vi "Vision Processing.vi"(4 "error in (no error)":errorcluster) -> ()   [LabVIEW 2015]
uses:
  Vision Support Code/Camera Types.ctl
  <vilib>/Rock Robotics/WPI/Camera/WPI_CameraImageSize.ctl
  <vilib>/Rock Robotics/WPI/Camera/WPI_CameraWhite Balance Values.ctl
  <vilib>/Rock Robotics/WPI/Camera/WPI_CameraExposure Values.ctl
  <vilib>/Rock Robotics/WPI/Camera/WPI_CameraFrameRate.ctl
  Robot Global Data.vi
  <vilib>/vision/NI_Vision_Development_Module.lvlib
panel:
  in  "Image Size":T1=enum."320x240"
  in  "Image Size 2":T1=enum."320x240"
  out "Highest Aspect":dbl=-1.0
  out "Target 2":bool
  out "Target 1":bool
  in  "Center Threshold":dbl=0.1
  out "Target 0":bool
  out "Highest Avg Score":dbl
  in  "Min Score Threshold":i32=75
  out "Detected Targets":T2(array[cluster]) {"Normalized Rect"."Numeric 5" format="%#_2g"; "Normalized Rect"."Numeric 3" format="%#_2g"; "Normalized Rect"."Numeric 2" format="%#_2g"; "Normalized Rect"."Numeric" format="%#_2g"}
  out "Sorted Particle Scores":T3(array[cluster]) {"Moment Factor" format="%#_3g"; "Aspect Ratio" format="%#_3g"; "Area to CH" format="%#_3g"; "X" format="%#_3g"; "Y" format="%#_3g"}
  in  "Display Original":bool
  in  "Display Mask":bool
  out "fps":dbl
  in  "Emphasize Limit Tests":bool
  in  "Camera Type":T4=enum."MS HD3000 square"
  in  "Aspect Fudge Factor":dbl=1.0
  in  "Score Threshold":dbl=75.0
  out "ms to process":u32
  out "Qualified Particles":i32
  in  "LED Color":T5={"Hue"={17.898766599709568, 122.67388403082947}, "Sat"={24.285714285714295, 255.0}, "Val"={145.71428571428572, 255.0}} {"Hue" scale=0.0..255.0 scale format="%#_3g"}
  out "Masked":T6(plugin-control)
  out "Original Image":T6(plugin-control)
  # "This is only the initial camera size.\nOther camera setup is done\non the diagram. Notice it is set\nonce before the loop but can be\nupdated within the loop if needed."
  # "Instructions:\nUse LED Color to threshold and build particles. Adjust calibration if needed.\nDisplays are very useful for debugging, but will slow down execution, so you\nmay want to disable once working.\nAnnotations show the rectangle and the scores from top to bottom.\nChange camera setting on diagram."
  # "Density Profile"
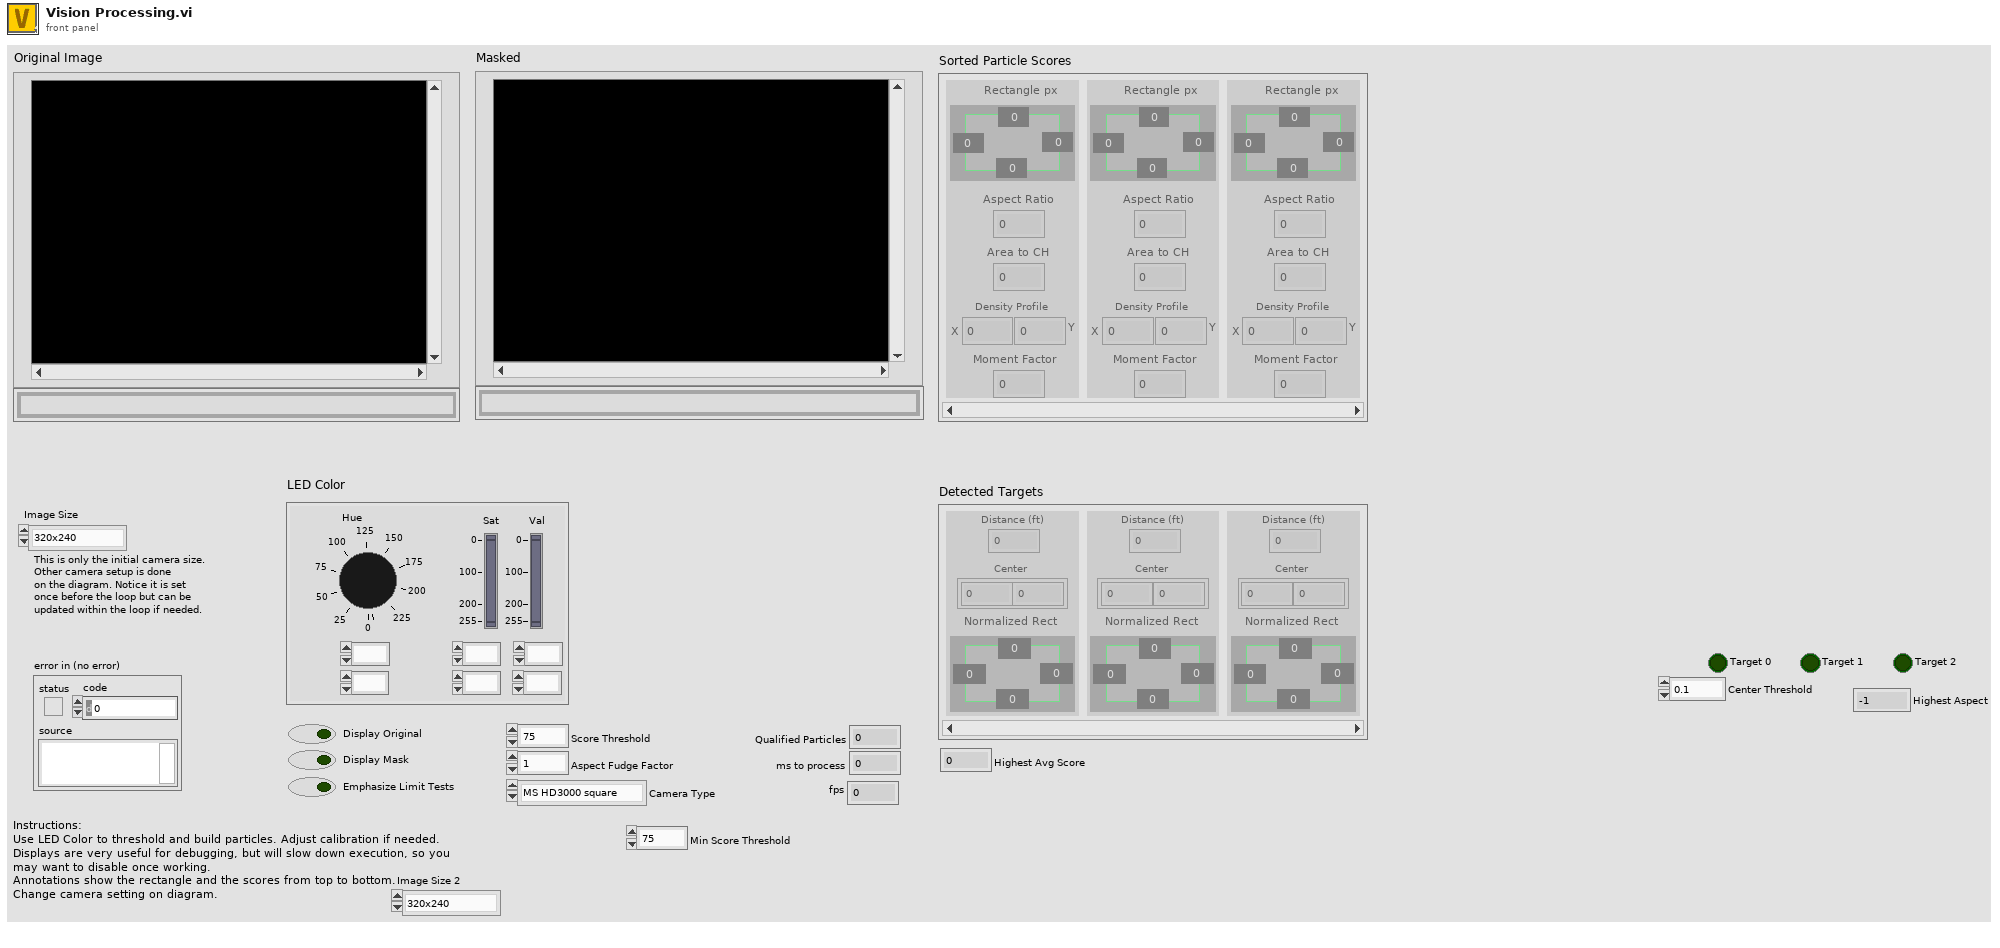
[diagram p1: front panel]
types:
  T1 = typedef "WPI_CameraImageSize.ctl" = enum16{"640x480", "320x240", "160x120", "Custom"}
  T2 = cluster{"Distance (ft)":dbl, "Center":cluster{dbl, dbl}, "Normalized Rect":cluster{"Numeric":dbl, "Numeric 2":dbl, "Numeric 3":dbl, "Numeric 5":dbl}}[]
  T3 = cluster{"Rectangle px":cluster{"Numeric":dbl, "Numeric 2":dbl, "Numeric 3":dbl, "Numeric 5":dbl}, "Aspect Ratio":dbl, "Area to CH":dbl, "X":dbl, "Y":dbl, "Moment Factor":dbl}[]
  T4 = typedef "Camera Types.ctl" = enum16{"206", "1011", "1013", "MS HD3000 square", "MS HD3000 640x480"}
  T5 = cluster{"Hue":cluster{dbl, dbl}, "Sat":cluster{dbl, dbl}, "Val":cluster{dbl, dbl}}
  T6 = typedef "IMAQ Image.ctl" = refnum<image>
  T7 = typedef "WPI_CameraFrameRate.ctl" = u32
  T8 = typedef "WPI_CameraWhite Balance Values.ctl" = enum16{"Auto", "Fixed indoor", "Fixed outdoor 1", "Fixed outdoor 2", "Fixed fluorescent 1", "Fixed fluorescent 2", "Hold current", "Custom"}
  T9 = typedef "WPI_CameraExposure Values.ctl" = enum16{"Auto", "Flicker-free 50 Hz", "Flicker-free 60 Hz", "Hold current", "Custom"}
  T10 = typedef "Particle Parameters" = i32
  T11 = typedef "Image Type" = u32
  T12 = typedef "WPI_CameraDevRef.ctl" = cluster{"Camera Address":string, "CameraStatus":errorcluster}
  T13 = cluster{"Bounding box":cluster{"left":dbl, "top":dbl, "right":dbl, "bottom":dbl}, "Aspect Ratio":dbl, "Area to CH":dbl, "X Mask":dbl, "Y Mask":dbl, "Moment":dbl}[]
  T14 = cluster{"Rectangle":cluster{"Numeric":dbl, "Numeric 2":dbl, "Numeric 3":dbl, "Numeric 5":dbl}, "L":dbl, "Area to CH":dbl, "X":dbl, "Y":dbl, "Moment Factor":dbl}[]
  T15 = cluster{"Sorted Scores[0]":cluster{"Rectangle":cluster{"Numeric":dbl, "Numeric 2":dbl, "Numeric 3":dbl, "Numeric 5":dbl}, "L":dbl, "Area to CH":dbl, "X":dbl, "Y":dbl, "Moment Factor":dbl}, "Sorted Scores[1]":cluster{"Rectangle":cluster{"Numeric":dbl, "Numeric 2":dbl, "Numeric 3":dbl, "Numeric 5":dbl}, "L":dbl, "Area to CH":dbl, "X":dbl, "Y":dbl, "Moment Factor":dbl}, "Sorted Scores[2]":cluster{"Rectangle":cluster{"Numeric":dbl, "Numeric 2":dbl, "Numeric 3":dbl, "Numeric 5":dbl}, "L":dbl, "Area to CH":dbl, "X":dbl, "Y":dbl, "Moment Factor":dbl}, "Sorted Scores[3]":cluster{"Rectangle":cluster{"Numeric":dbl, "Numeric 2":dbl, "Numeric 3":dbl, "Numeric 5":dbl}, "L":dbl, "Area to CH":dbl, "X":dbl, "Y":dbl, "Moment Factor":dbl}, "Sorted Scores[4]":cluster{"Rectangle":cluster{"Numeric":dbl, "Numeric 2":dbl, "Numeric 3":dbl, "Numeric 5":dbl}, "L":dbl, "Area to CH":dbl, "X":dbl, "Y":dbl, "Moment Factor":dbl}, "Sorted Scores[5]":cluster{"Rectangle":cluster{"Numeric":dbl, "Numeric 2":dbl, "Numeric 3":dbl, "Numeric 5":dbl}, "L":dbl, "Area to CH":dbl, "X":dbl, "Y":dbl, "Moment Factor":dbl}, "Sorted Scores[6]":cluster{"Rectangle":cluster{"Numeric":dbl, "Numeric 2":dbl, "Numeric 3":dbl, "Numeric 5":dbl}, "L":dbl, "Area to CH":dbl, "X":dbl, "Y":dbl, "Moment Factor":dbl}, "Sorted Scores[7]":cluster{"Rectangle":cluster{"Numeric":dbl, "Numeric 2":dbl, "Numeric 3":dbl, "Numeric 5":dbl}, "L":dbl, "Area to CH":dbl, "X":dbl, "Y":dbl, "Moment Factor":dbl}, "Sorted Scores[8]":cluster{"Rectangle":cluster{"Numeric":dbl, "Numeric 2":dbl, "Numeric 3":dbl, "Numeric 5":dbl}, "L":dbl, "Area to CH":dbl, "X":dbl, "Y":dbl, "Moment Factor":dbl}}
  T16 = cluster{"Found Targets[0]":cluster{"Distance (ft)":dbl, "Center":cluster{dbl, dbl}, "Normalized Rect":cluster{"Numeric":dbl, "Numeric 2":dbl, "Numeric 3":dbl, "Numeric 5":dbl}}, "Found Targets[1]":cluster{"Distance (ft)":dbl, "Center":cluster{dbl, dbl}, "Normalized Rect":cluster{"Numeric":dbl, "Numeric 2":dbl, "Numeric 3":dbl, "Numeric 5":dbl}}, "Found Targets[2]":cluster{"Distance (ft)":dbl, "Center":cluster{dbl, dbl}, "Normalized Rect":cluster{"Numeric":dbl, "Numeric 2":dbl, "Numeric 3":dbl, "Numeric 5":dbl}}, "Found Targets[3]":cluster{"Distance (ft)":dbl, "Center":cluster{dbl, dbl}, "Normalized Rect":cluster{"Numeric":dbl, "Numeric 2":dbl, "Numeric 3":dbl, "Numeric 5":dbl}}, "Found Targets[4]":cluster{"Distance (ft)":dbl, "Center":cluster{dbl, dbl}, "Normalized Rect":cluster{"Numeric":dbl, "Numeric 2":dbl, "Numeric 3":dbl, "Numeric 5":dbl}}, "Found Targets[5]":cluster{"Distance (ft)":dbl, "Center":cluster{dbl, dbl}, "Normalized Rect":cluster{"Numeric":dbl, "Numeric 2":dbl, "Numeric 3":dbl, "Numeric 5":dbl}}, "Found Targets[6]":cluster{"Distance (ft)":dbl, "Center":cluster{dbl, dbl}, "Normalized Rect":cluster{"Numeric":dbl, "Numeric 2":dbl, "Numeric 3":dbl, "Numeric 5":dbl}}, "Found Targets[7]":cluster{"Distance (ft)":dbl, "Center":cluster{dbl, dbl}, "Normalized Rect":cluster{"Numeric":dbl, "Numeric 2":dbl, "Numeric 3":dbl, "Numeric 5":dbl}}, "Found Targets[8]":cluster{"Distance (ft)":dbl, "Center":cluster{dbl, dbl}, "Normalized Rect":cluster{"Numeric":dbl, "Numeric 2":dbl, "Numeric 3":dbl, "Numeric 5":dbl}}}
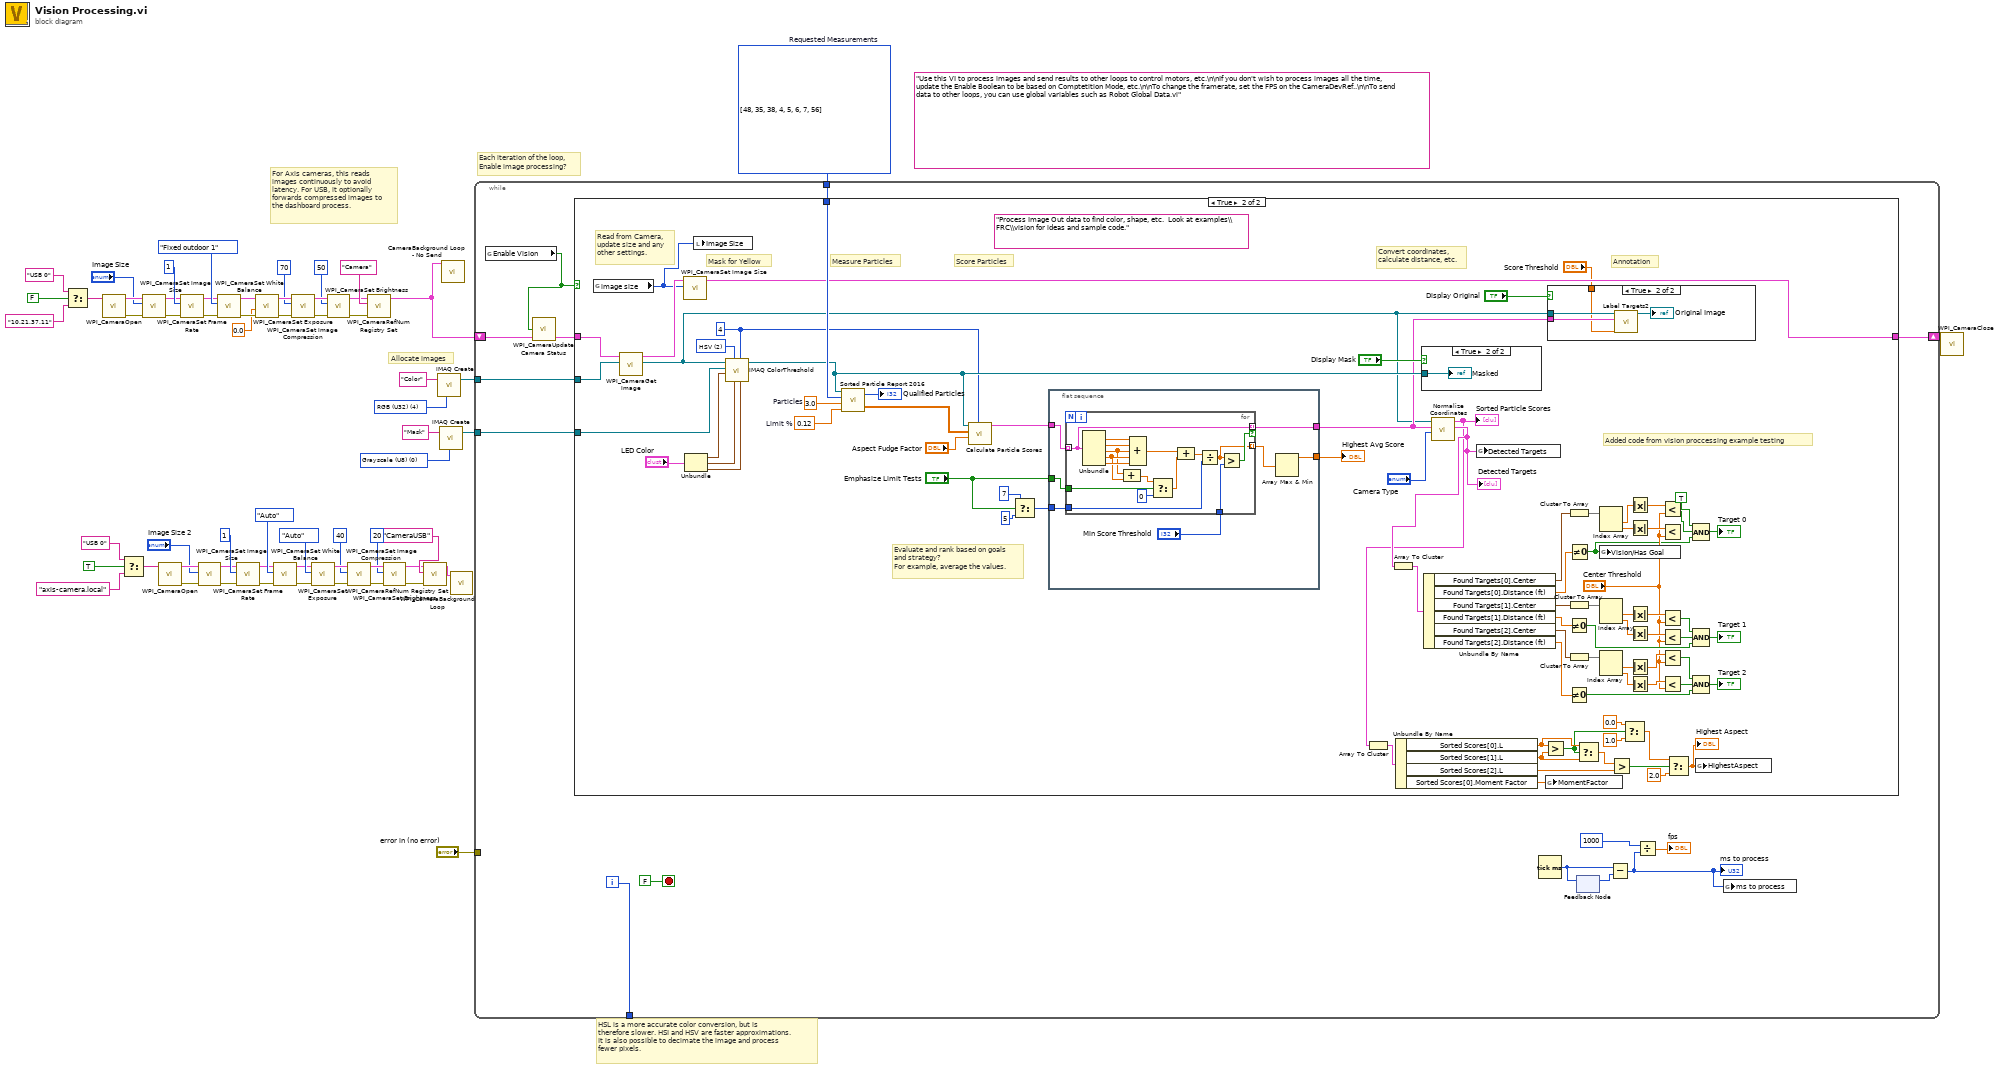
[diagram p0: block diagram]
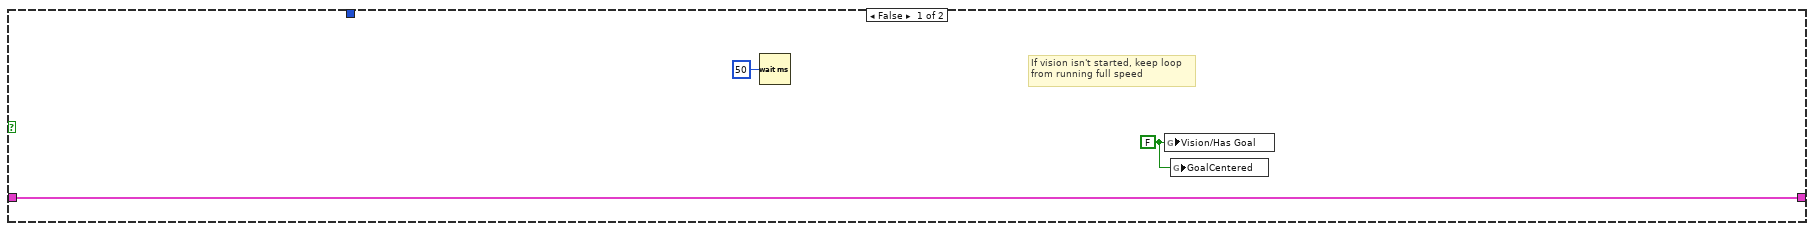
[diagram p2: hidden frame]
diagram:
  (unwired) "Use this VI to process images and send results to other loops to control motors, etc.\n\nIf you don't wish to process images all the time, update the Enable Boolean to be based on Comptetition Mode, etc.\n\nTo change the framerate, set the FPS on the CameraDevRef..\n\nTo send data to other loops, you can use global variables such as Robot Global Data.vi"
  w55 = T10[] [48, 35, 38, 4, 5, 6, 7, 56] items=["Center of Mass X", "Center of Mass Y", "First Pixel X", "First Pixel Y", "Bounding Rect Left", "Bounding Rect Top", "Bounding Rect Right", "Bounding Rect Bottom", "Max Feret Diameter Start X", "Max Feret Diameter Start Y", "Max Feret Diameter End X", "Max Feret Diameter End Y", "Max Horiz. Segment Length Left", "Max Horiz. Segment Length Right", "Max Horiz. Segment Length Row", "-", "Bounding Rect Width", "Bounding Rect Height", "Bounding Rect Diagonal", "Perimeter", "Convex Hull Perimeter", "Holes' Perimeter", "Max Feret Diameter", "Equivalent Ellipse Major Axis", "Equivalent Ellipse Minor Axis", "Equivalent Ellipse Minor Axis (Feret)", "Equivalent Rect Long Side", "Equivalent Rect Short Side", "Equivalent Rect Diagonal", "Equivalent Rect Short Side (Feret)", "Average Horiz. Segment Length", "Average Vert. Segment Length", "Hydraulic Radius", "Waddel Disk Diameter", "-", "Area", "Holes' Area", "Particle & Holes' Area", "Convex Hull Area", "Image Area", "-", "Number of Holes", "Number of Horiz. Segments", "Number of Vert. Segments", "-", "Orientation", "Max Feret Diameter Orientation", "-", "% Area/Image Area", "% Area/(Particle & Holes' Area)", "Ratio of Equivalent Ellipse Axes", "Ratio of Equivalent Rect Sides", "-", "Elongation Factor", "Compactness Factor", "Heywood Circularity Factor", "Type Factor", "-", "Sum X", "Sum Y", "Sum XX", "Sum XY", "Sum YY", "Sum XXX", "Sum XXY", "Sum XYY", "Sum YYY", "-", "Moment of Inertia XX", "Moment of Inertia XY", "Moment of Inertia YY", "Moment of Inertia XXX", "Moment of Inertia XXY", "Moment of Inertia XYY", "Moment of Inertia YYY", "Norm. Moment of Inertia XX", "Norm. Moment of Inertia XY", "Norm. Moment of Inertia YY", "Norm. Moment of Inertia XXX", "Norm. Moment of Inertia XXY", "Norm. Moment of Inertia XYY", "Norm. Moment of Inertia YYY", "Hu Moment 1", "Hu Moment 2", "Hu Moment 3", "Hu Moment 4", "Hu Moment 5", "Hu Moment 6", "Hu Moment 7"]  # Requested Measurements
  w58 = T11 0 items=["Grayscale (U8)", "Grayscale (I16)", "Grayscale (SGL)", "Complex (CSG)", "RGB (U32)", "HSL (U32)", "RGB (U64)", "Grayscale (U16)"] ("Image Type")
  w60 = T11 4 items=["Grayscale (U8)", "Grayscale (I16)", "Grayscale (SGL)", "Complex (CSG)", "RGB (U32)", "HSL (U32)", "RGB (U64)", "Grayscale (U16)"] ("Image Type")
  # "Each iteration of the loop,\nEnable image processing?"
  # "HSL is a more accurate color conversion, but is\ntherefore slower. HSI and HSV are faster approximations.\nIt is also possible to decimate the image and process\nfewer pixels."
  # "For Axis cameras, this reads\nimages continuously to avoid\nlatency. For USB, it optionally\nforwards compressed images to\nthe dashboard process."
  # "Allocate images"
  n1 = Select(t="USB 0" ("format string"), s=FALSE ("dot notation? (F)"), f="10.21.37.11" ("format string")) -> (s? t:f=w26:string)
  n2 = call <vilib>:"WPI_CameraOpen.vi"("Camera Address"=w26) -> ("error out"=w15:errorcluster, "CameraDevRef"=w14:T12)  [unwired: 1 in, 8 out]
  n3 = Select(t="USB 0" ("format string"), s=TRUE ("dot notation? (F)"), f="axis-camera.local" ("format string")) -> (s? t:f=w52:string)
  n4 = call <vilib>:"WPI_CameraSet Image Size.vi"("error in (no error)"=w15, "Image Size"="Image Size", "CameraDevRef"=w14) -> ("error out"=w16:errorcluster, "CameraDevRef Out"=w13:T12)  [unwired: 1 in, 6 out]
  n5 = call <vilib>:"WPI_CameraOpen.vi"("Camera Address"=w52) -> ("error out"=w40:errorcluster, "CameraDevRef"=w39:T12)  [unwired: 1 in, 8 out]
  n6 = call <vilib>:"WPI_CameraSet Frame Rate.vi"("error in (no error)"=w16, "Frame Rate (fps)"=T7 1, "CameraDevRef"=w13) -> ("error out"=w17:errorcluster, "CameraDevRef Out"=w11:T12)  [unwired: 7 out]
  n7 = call <vilib>:"WPI_CameraSet Image Size.vi"("error in (no error)"=w40, "Image Size"="Image Size 2", "CameraDevRef"=w39) -> ("error out"=w41:errorcluster, "CameraDevRef Out"=w38:T12)  [unwired: 1 in, 6 out]
  n8 = call <vilib>:"WPI_CameraSet White Balance.vi"("error in (no error)"=w17, "White Balance"=WPI_CameraWhite_Balance_Values."Fixed outdoor 1", "CameraDevRef"=w11) -> ("error out"=w18:errorcluster, "CameraDevRef Out"=w12:T12)  [unwired: 1 in, 6 out]
  n9 = call <vilib>:"WPI_CameraSet Frame Rate.vi"("error in (no error)"=w41, "Frame Rate (fps)"=T7 1, "CameraDevRef"=w38) -> ("error out"=w42:errorcluster, "CameraDevRef Out"=w36:T12)  [unwired: 7 out]
  n10 = call <vilib>:"WPI_CameraSet Exposure.vi"("error in (no error)"=w18, "Exposure (%)"=0.0, "CameraDevRef"=w12) -> ("error out"=w19:errorcluster, "CameraDevRef Out"=w9:T12)  [unwired: 1 in, 6 out]
  n11 = call <vilib>:"WPI_CameraSet White Balance.vi"("error in (no error)"=w42, "White Balance"=WPI_CameraWhite_Balance_Values."Auto", "CameraDevRef"=w36) -> ("error out"=w43:errorcluster, "CameraDevRef Out"=w37:T12)  [unwired: 1 in, 6 out]
  n12 = call <vilib>:"WPI_CameraSet Image Compression.vi"("error in (no error)"=w19, "Compression"=70, "CameraDevRef"=w9) -> ("error out"=w20:errorcluster, "CameraDevRef Out"=w10:T12)  [unwired: 7 out]
  n13 = call <vilib>:"WPI_CameraSet Exposure.vi"("error in (no error)"=w43, "Exposure"=WPI_CameraExposure_Values."Auto", "CameraDevRef"=w37) -> ("error out"=w44:errorcluster, "CameraDevRef Out"=w34:T12)  [unwired: 1 in, 6 out]
  n14 = call <vilib>:"WPI_CameraSet Brightness.vi"("error in (no error)"=w20, "Brightness"=50, "CameraDevRef"=w10) -> ("error out"=w21:errorcluster, "CameraDevRef Out"=w4:T12)  [unwired: 7 out]
  n15 = call <vilib>:"WPI_CameraSet Image Compression.vi"("error in (no error)"=w44, "Compression"=40, "CameraDevRef"=w34) -> ("error out"=w45:errorcluster, "CameraDevRef Out"=w35:T12)  [unwired: 7 out]
  n16 = call <vilib>:"WPI_CameraRefNum Registry Set.vi"("error in (no error)"=w21, "refnum name"="Camera", "CameraDevRef"=w4) -> ("CameraDevRef"=w3:T12)  [unwired: 1 in, 7 out]
  n17 = call <vilib>:"WPI_CameraSet Brightness.vi"("error in (no error)"=w45, "Brightness"=20, "CameraDevRef"=w35) -> ("error out"=w46:errorcluster, "CameraDevRef Out"=w28:T12)  [unwired: 7 out]
  n18 = call <vilib>:"WPI_CameraRefNum Registry Set.vi"("error in (no error)"=w46, "refnum name"="CameraUSB", "CameraDevRef"=w28) -> ("CameraDevRef"=w27:T12)  [unwired: 1 in, 7 out]
  n19 = call "IMAQ Create"("Image Name"="Color", "Image Type"=w60) -> ("New Image"=w59:T6)  [unwired: 2 in, 2 out]
  n20 = call "IMAQ Create"("Image Name"="Mask", "Image Type"=w58) -> ("New Image"=w56:T6)  [unwired: 2 in, 2 out]
  n21 = call "CameraBackground Loop - No Send.vi"("CameraDevRef"=w3) -> ()  [unwired: 11 in]
  n22 = call <vilib>:"WPI_CameraBackground Loop.vi"("CameraDevRef"=w27) -> ()  [unwired: 11 in]
  n23 = while {
    tunnel: w59 -> [w70]
    tunnel: w56 -> [w74]
    tunnel: w55 -> [w73]
    tunnel: "error in (no error)" -> [_]
    tunnel: [w69] -> _
    shift-right: [w66] -> w53
    shift-left: w3 -> [w68]
    i -> [w69]
    stop <- FALSE stop-if-true
    n24 = global read "Robot Global Data.vi" "Enable Vision"() -> (w62:bool)
    n25 = call <vilib>:"WPI_CameraUpdate Camera Status.vi"("CameraDevRef In"=w68, "Enable Vision"=w62) -> ("CameraDevRef Out"=w67:T12)  [unwired: 3 in]
    n26 = case shown="True" w62 {
      tunnel: w74 -> [_ w159]
      tunnel: w73 -> [_ w154]
      tunnel: w67 -> [w77 w150]
      tunnel: w70 -> [_ w149]
      tunnel: [w77 w147] -> w66
      frame False {
        w76 = FALSE ("Vision/Has Goal")
        # "If vision isn't started, keep loop\nfrom running full speed"
        n27 = Wait (ms)(milliseconds to wait=u32 50) -> ()  [unwired: 1 out]
        n28 = global write "Robot Global Data.vi" "Vision/Has Goal"(w76) -> ()
        n29 = global write "Robot Global Data.vi" "GoalCentered"(w76) -> ()
      }
      frame True {
        w132 = 4 ("Replace Value")
        w144 = u16 2 items=["RGB", "HSL", "HSV", "HSI"] ("Color Mode")
        (unwired) "Process Image Out data to find color, shape, etc.  Look at examples\\FRC\\vision for ideas and sample code."
        w151 = 0.12  # Limit %
        w153 = 3.0  # Particles
        # "Added code from vision proccessing example testing"
        # "Evaluate and rank based on goals\nand strategy?\nFor example, average the values."
        # "Read from Camera,\nupdate size and any\nother settings."
        # "Measure Particles"
        # "Convert coordinates,\ncalculate distance, etc."
        # "Annotation"
        # "Score Particles"
        # "Mask for Yellow"
        n30 = global read "Robot Global Data.vi" "image size"() -> (w80:T1)
        n31 = call <vilib>:"WPI_CameraGet Image.vi"("Image"=w149, "CameraDevRef"=w150) -> ("Image Out"=w81:T6, "CameraDevRef Out"=w148:T12)  [unwired: 7 in, 1 out]
        n32 = call <vilib>:"WPI_CameraSet Image Size.vi"("Image Size"=w80, "CameraDevRef"=w148) -> ("CameraDevRef Out"=w147:T12)  [unwired: 2 in, 7 out]
        n33 = Unbundle("LED Color") -> ("Hue"=w158:cluster{dbl, dbl}, "Sat"=w157:cluster{dbl, dbl}, "Val"=w156:cluster{dbl, dbl})
        n34 = local write "Image Size"(w80) -> ()
        n35 = call "IMAQ ColorThreshold"("Blue or Luma or Val or Inten Range"=w156, "Replace Value"=w132, "Green or Sat Range"=w157, "Color Mode"=w144, "Red or Hue Range"=w158, "Image Dst"=w159, "Image Src"=w81) -> ("Image Dst Out"=w143:T6)  [unwired: 3 in, 1 out]
        n36 = call "Sorted Particle Report 2016.vi"("Min Area Size %"=w151, "Particle Count Limit"=w153, "Pixel Measurements"=w154, "Image in"=w143) -> ("Sorted Data"=w142:dbl[][], "Particles"=→"Qualified Particles":i32)
        n37 = call "Calculate Particle Scores.vi"("Pixel Value"=w132, "Aspect Fudge Factor"="Aspect Fudge Factor", "Sorted Data"=w142, "Image in"=w143) -> ("Scores"=w140:T13)  [unwired: 7 in]
        n38 = Select(t=7, s="Emphasize Limit Tests", f=5) -> (s? t:f=w137:i32)
        n39 = flat-sequence {
          tunnel: w140 -> [w170]
          tunnel: w137 -> [w168]
          tunnel: [w171] -> w136
          tunnel: [w165] -> w134
          tunnel: "Emphasize Limit Tests" -> [w169]
          frame #0 {
            n40 = for {
              tunnel: w170 -> [w185] mode=indexing
              tunnel: [w185] -> w165 mode=indexing if=w184
              tunnel: [w183] -> w166 mode=indexing
              tunnel: w168 -> [w182]
              tunnel: "Min Score Threshold" -> [w181]
              tunnel: w169 -> [w174]
              n41 = Unbundle(w185) -> ("Aspect Ratio"=w187:dbl, "Area to CH"=w186:dbl, "X Mask"=w176:dbl, "Y Mask"=w177:dbl, "Moment"=w178:dbl)  [unwired: 1 out]
              n42 = Compound Arithmetic op=ADD(w176, w177) -> (w175:dbl)
              n43 = Compound Arithmetic op=ADD(w187, w186, w176, w177, w178) -> (w180:dbl)
              n44 = Select(t=w175, s=w174, f=0) -> (s? t:f=w173:dbl)
              n45 = Compound Arithmetic op=ADD(w180, w173) -> (w179:dbl)
              n46 = Divide(x=w179, y=w182) -> (x/y=w183:dbl)
              n47 = Greater?(x=w183, y=w181) -> (0:w184:bool)
            }
            n48 = Array Max & Min(array=w166) -> (max value=w171:dbl)  [unwired: 3 out]
          }
        }
        n49 = case shown="True" "Display Mask" {
          tunnel: w143 -> [_ w164]
          frame False {
          }
          frame True {
            "Masked" <- w164
          }
        }
        n50 = call "Normalize Coordinates.vi"("Camera Type"="Camera Type", "Targets"=w134, "Image in"=w81) -> ("Found Targets"=w88:T2, "Sorted Scores"=w87:T14)  [unwired: 7 in]
        "Sorted Particle Scores" <- w87
        "Detected Targets" <- w88
        n51 = Array To Cluster(array=w87) -> (cluster=w99:T15)
        n52 = Array To Cluster(array=w88) -> (cluster=w85:T16)
        n53 = Unbundle By Name(w99) -> ("Sorted Scores[0].L"=w94:dbl, "Sorted Scores[1].L"=w93:dbl, "Sorted Scores[2].L"=w95:dbl, "Sorted Scores[0].Moment Factor"=w79:dbl)
        n54 = Unbundle By Name(w85) -> ("Found Targets[0].Center"=w130:cluster{dbl, dbl}, "Found Targets[0].Distance (ft)"=w123:dbl, "Found Targets[1].Center"=w114:cluster{dbl, dbl}, "Found Targets[1].Distance (ft)"=w113:dbl, "Found Targets[2].Center"=w103:cluster{dbl, dbl}, "Found Targets[2].Distance (ft)"=w102:dbl)
        n55 = global write "Robot Global Data.vi" "Detected Targets"(w88) -> ()
        n56 = Greater?(x=w94, y=w93) -> (0:w92:bool)
        n57 = global write "Robot Global Data.vi" "MomentFactor"(w79) -> ()
        n58 = case shown="True" "Display Original" {
          tunnel: w81 -> [_ w163]
          tunnel: w134 -> [_ w161]
          tunnel: "Score Threshold" -> [_ w160]
          frame False {
          }
          frame True {
            n59 = call "Label Targets2.vi"("Score Threshold"=w160, "Targets"=w161, "Image in"=w163) -> ("Image out"=→"Original Image":T6)  [unwired: 8 in]
          }
        }
        n60 = Cluster To Array(cluster=w130) -> (array=w129:dbl[])
        n61 = Cluster To Array(cluster=w114) -> (array=w122:dbl[])
        n62 = Not Equal To 0?(x=w113) -> (x != 0?=w115:bool)
        n63 = Cluster To Array(cluster=w103) -> (array=w111:dbl[])
        n64 = Not Equal To 0?(x=w102) -> (x != 0?=w104:bool)
        n65 = Not Equal To 0?(x=w123) -> (x != 0?=w86:bool)
        n66 = Select(t=w94, s=w92, f=w93) -> (s? t:f=w90:dbl)
        n67 = Index Array(array=w129) -> (element #1=w127:dbl, element #2=w128:dbl)  [unwired: 2 in]
        n68 = global write "Robot Global Data.vi" "Vision/Has Goal"(w86) -> ()
        n69 = Index Array(array=w122) -> (element #1=w120:dbl, element #2=w121:dbl)  [unwired: 2 in]
        n70 = Index Array(array=w111) -> (element #1=w109:dbl, element #2=w110:dbl)  [unwired: 2 in]
        n71 = Greater?(x=w90, y=w95) -> (0:w96:bool)
        n72 = Select(t=0.0, s=w92, f=1.0) -> (s? t:f=w89:dbl)
        n73 = Absolute Value(x=w127) -> (abs(x)=w126:dbl)
        n74 = Absolute Value(x=w128) -> (abs(x)=w125:dbl)
        n75 = Absolute Value(x=w120) -> (abs(x)=w119:dbl)
        n76 = Absolute Value(x=w121) -> (abs(x)=w118:dbl)
        n77 = Absolute Value(x=w109) -> (abs(x)=w108:dbl)
        n78 = Absolute Value(x=w110) -> (abs(x)=w107:dbl)
        n79 = Less?(x=w126, y="Center Threshold") -> (x < y?=w124:bool)
        n80 = Less?(x=w125, y="Center Threshold") -> ()  [unwired: 1 out]
        n81 = Less?(x=w119, y="Center Threshold") -> (x < y?=w117:bool)
        n82 = Less?(x=w118, y="Center Threshold") -> (x < y?=w116:bool)
        n83 = Less?(x=w108, y="Center Threshold") -> (x < y?=w106:bool)
        n84 = Less?(x=w107, y="Center Threshold") -> (x < y?=w105:bool)
        n85 = Select(t=w89, s=w96, f=2.0) -> (s? t:f=w82:dbl)
        "Highest Aspect" <- w82
        n86 = Compound Arithmetic op=AND(w124, TRUE ("value"), w86) -> (→"Target 0":bool)
        n87 = Compound Arithmetic op=AND(w117, w116, w115) -> (→"Target 1":bool)
        n88 = Compound Arithmetic op=AND(w106, w105, w104) -> (→"Target 2":bool)
        n89 = global write "Robot Global Data.vi" "HighestAspect"(w82) -> ()
        "Highest Avg Score" <- w136
      }
    }
    n90 = Tick Count (ms)() -> (millisecond timer value=w71:u32)
    n91 = feedback-in #1(w71) -> ()
    n92 = feedback #1() -> (w72:u32)  [unwired: 1 in]
    n93 = Subtract(x=w71, y=w72) -> (x-y=w65:u32)
    "ms to process" <- w65
    n94 = Divide(x=1000 ("Brightness"), y=w65) -> (x/y=→"fps":dbl)
    n95 = global write "Robot Global Data.vi" "ms to process"(w65) -> ()
  }
  n96 = call <vilib>:"WPI_CameraClose.vi"("CameraDevRef"=w53) -> ()  [unwired: 1 in, 10 out]
